vi "Timeout.vi"(8 "error in (no error)":errorcluster, 9 "Timeout (ms)":i32=5000, 10 "Start Time":u32) -> (0 "error out":errorcluster, 4 "Timeout?":bool)   [LabVIEW 2014]
uses:
  <vilib>/Utility/error.llb/Error Cluster From Error Code.vi
  <vilib>/ErrorRing/Error Ring.xnode
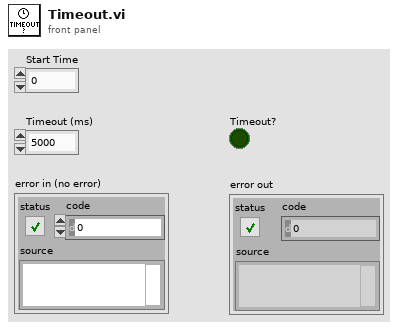
[diagram p1: front panel]
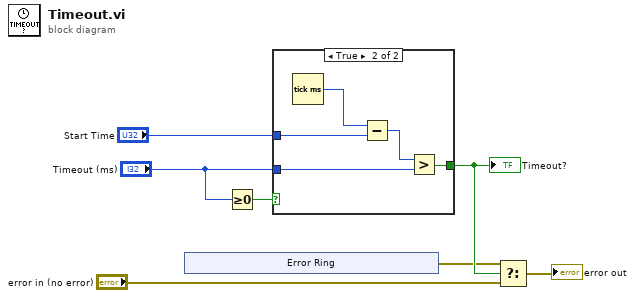
[diagram p0: block diagram]
diagram:
  n1 = xnode "Error Ring"() -> ("error out"=w3:errorcluster)
  n2 = Greater Or Equal To 0?(x="Timeout (ms)") -> (x >= 0?=w7:bool)
  n3 = case shown="True" w7 {
    tunnel: "Timeout (ms)" -> [_ w9]
    tunnel: "Start Time" -> [_ w11]
    tunnel: [_ w8] -> w4
    frame False {
    }
    frame True {
      n4 = Tick Count (ms)() -> (millisecond timer value=w12:u32)
      n5 = Subtract(x=w12, y=w11) -> (x-y=w10:u32)
      n6 = Greater?(x=w10, y=w9) -> (0:w8:bool)
    }
  }
  "Timeout?" <- w4
  n7 = Select(t=w3, s=w4, f="error in (no error)") -> (s? t:f=→"error out":errorcluster)
